vi "AutoCal.vi"(9 "Std Devs":dbl=1.0, 10 "Target Color":enum16{"Red", "Green", "Blue"}(ring), 11 "Color Image":T1) -> (1 "Luminance Info":T2, 2 "Saturation Info":T2, 3 "Hue Info":T2, 5 "Number of Particles":i32)   [LabVIEW 2013]
uses:
  <vilib>/vision/Image Controls.llb/IMAQ Image.ctl
  <vilib>/vision/NI_Vision_Development_Module.lvlib
panel:
  in  "Manual":bool
  out "Original":T1(plugin-control)
  out "Lum Std Dev":sgl format="%.2f"
  out "Lum Mean":sgl format="%.2f"
  out "Sat Std Dev":sgl format="%.2f"
  out "Sat Mean":sgl format="%.2f"
  out "Hue Std Dev":sgl format="%.2f"
  out "Hue Mean":sgl format="%.2f"
  out "Waveform Graph 2":T3(graph)
  out "Search Color Standard  Dev":sgl format="%.2f"
  out "Search Color Mean":sgl format="%.2f"
  out "Waveform Graph":T4(graph)
  out "Image":T1(plugin-control)
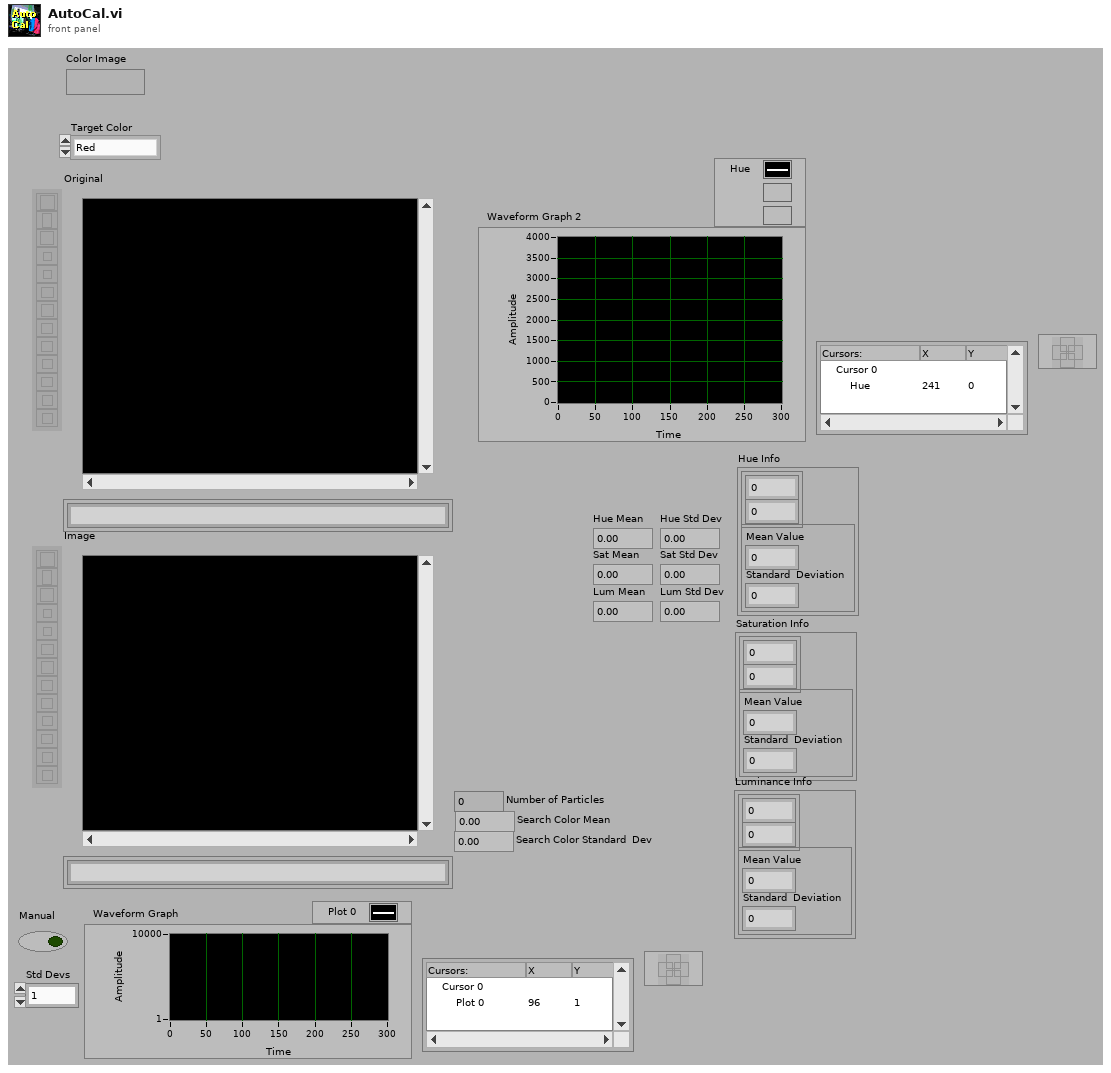
[diagram p1: front panel]
types:
  T1 = typedef "IMAQ Image.ctl" = refnum<image>
  T2 = cluster{cluster{sgl, sgl}, cluster{"Mean Value":sgl, "Standard  Deviation":sgl}}
  T3 = cluster{"Starting Value":sgl, "Incremental Value":sgl, "Histogram":u32[]}[]
  T4 = cluster{"Starting Value":sgl, "Incremental Value":sgl, "Histogram":u32[]}
  T5 = cluster{"Mean Value":sgl, "Standard  Deviation":sgl}
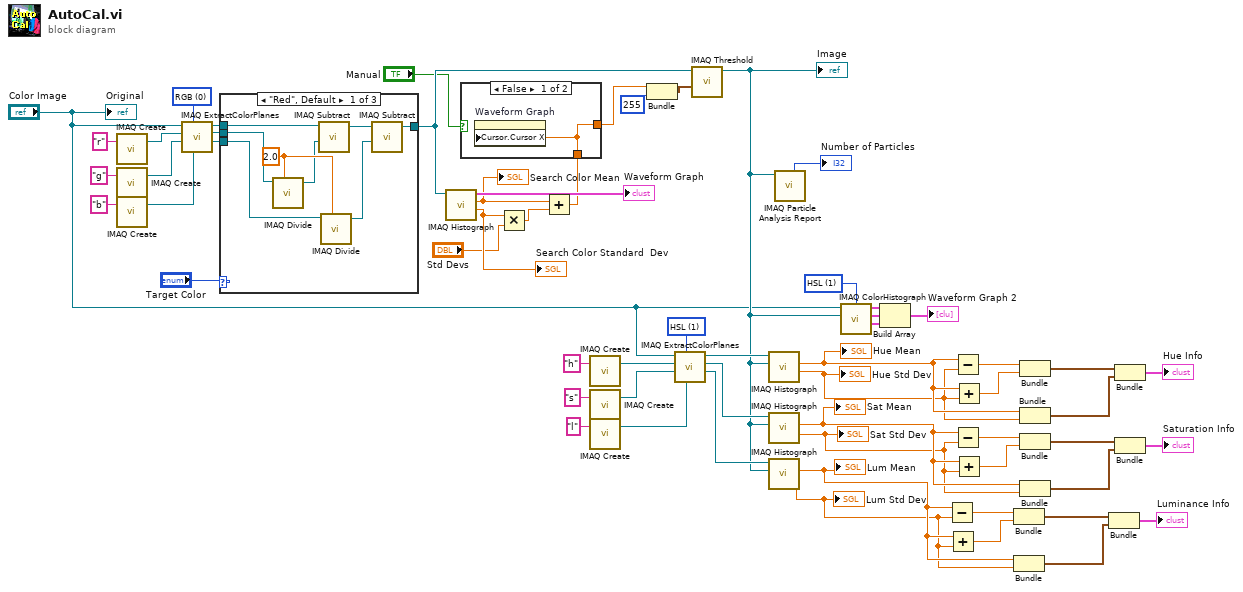
[diagram p0: block diagram]
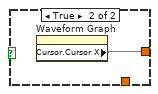
[diagram p2: hidden frame]
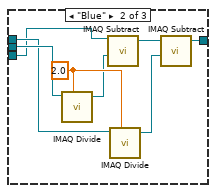
[diagram p3: hidden frame]
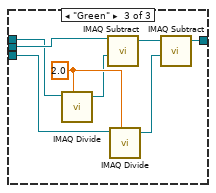
[diagram p4: hidden frame]
diagram:
  w42 = u16 1 items=["RGB", "HSL", "HSV", "HSI"] ("Color Mode")
  w47 = u16 1 items=["RGB", "HSL", "HSV", "HSI"] ("Color Mode")
  w55 = u16 0 items=["RGB", "HSL", "HSV", "HSI"] ("Color Mode")
  n1 = call "IMAQ Create"("Image Name"="r") -> ("New Image"=w58:T1)  [unwired: 3 in, 2 out]
  n2 = call "IMAQ Create"("Image Name"="g") -> ("New Image"=w57:T1)  [unwired: 3 in, 2 out]
  n3 = call "IMAQ Create"("Image Name"="b") -> ("New Image"=w56:T1)  [unwired: 3 in, 2 out]
  n4 = call "IMAQ ExtractColorPlanes"("Blue or Luma or Val or Inten Plane"=w56, "Color Mode"=w55, "Green or Sat Plane"=w57, "Red or Hue Plane"=w58, "Image Src"="Color Image") -> ("Blue or Luma or Val or Inten Plane out"=w53:T1, "Green or Sat Plane out"=w54:T1, "Red or Hue Plane out"=w52:T1)  [unwired: 1 in, 3 out]
  n5 = case shown="\"Red\", Default" "Target Color" {
    tunnel: w54 -> [w68 w72 w79]
    tunnel: w53 -> [w67 w70 w84]
    tunnel: w52 -> [w65 w71 w78]
    tunnel: [w62 w73 w80] -> w32
    frame "Red", Default {
      w66 = sgl 2.0 ("Constant")
      n6 = call "IMAQ Divide"("Image Src A"=w68, "Constant"=w66) -> ("Image Dst Out"=w64:T1)  [unwired: 4 in, 2 out]
      n7 = call "IMAQ Subtract"("Image Src A"=w65, "Image Src B"=w64) -> ("Image Dst Out"=w69:T1)  [unwired: 3 in, 3 out]
      n8 = call "IMAQ Divide"("Image Src A"=w67, "Constant"=w66) -> ("Image Dst Out"=w63:T1)  [unwired: 4 in, 2 out]
      n9 = call "IMAQ Subtract"("Image Src A"=w69, "Image Src B"=w63) -> ("Image Dst Out"=w62:T1)  [unwired: 3 in, 3 out]
    }
    frame "Blue" {
      w76 = sgl 2.0 ("Constant")
      n10 = call "IMAQ Divide"("Image Src A"=w72, "Constant"=w76) -> ("Image Dst Out"=w75:T1)  [unwired: 4 in, 2 out]
      n11 = call "IMAQ Subtract"("Image Src A"=w70, "Image Src B"=w75) -> ("Image Dst Out"=w77:T1)  [unwired: 3 in, 3 out]
      n12 = call "IMAQ Divide"("Image Src A"=w71, "Constant"=w76) -> ("Image Dst Out"=w74:T1)  [unwired: 4 in, 2 out]
      n13 = call "IMAQ Subtract"("Image Src A"=w77, "Image Src B"=w74) -> ("Image Dst Out"=w73:T1)  [unwired: 3 in, 3 out]
    }
    frame "Green" {
      w83 = sgl 2.0 ("Constant")
      n14 = call "IMAQ Divide"("Image Src A"=w78, "Constant"=w83) -> ("Image Dst Out"=w82:T1)  [unwired: 4 in, 2 out]
      n15 = call "IMAQ Subtract"("Image Src A"=w79, "Image Src B"=w82) -> ("Image Dst Out"=w85:T1)  [unwired: 3 in, 3 out]
      n16 = call "IMAQ Divide"("Image Src A"=w84, "Constant"=w83) -> ("Image Dst Out"=w81:T1)  [unwired: 4 in, 2 out]
      n17 = call "IMAQ Subtract"("Image Src A"=w85, "Image Src B"=w81) -> ("Image Dst Out"=w80:T1)  [unwired: 3 in, 3 out]
    }
  }
  n18 = call "IMAQ Histograph"("Image"=w32) -> ("Standard  Deviation"=w25:sgl, "Mean Value"=w48:sgl, "Histogram Graph"=→"Waveform Graph":T4)  [unwired: 4 in, 4 out]
  "Search Color Mean" <- w48
  "Search Color Standard  Dev" <- w25
  n19 = Multiply(x=w25, y="Std Devs") -> (x*y=w24:dbl)
  n20 = Add(x=w48, y=w24) -> (x+y=w26:dbl)
  n21 = case shown="False" "Manual" {
    tunnel: [w86 w87] -> w28
    tunnel: w26 -> [w86 _]
    frame False {
      n22 = property on="Waveform Graph" class="WFGraph (strict)"("Cursor.Cursor X"=w86) -> ()  [unwired: 2 in, 2 out]
    }
    frame True {
      n23 = property on="Waveform Graph" class="WFGraph (strict)"() -> ("Cursor.Cursor X"=w87:dbl)  [unwired: 2 in, 2 out]
    }
  }
  n24 = call "IMAQ Create"("Image Name"="h") -> ("New Image"=w38:T1)  [unwired: 3 in, 2 out]
  n25 = call "IMAQ Create"("Image Name"="s") -> ("New Image"=w37:T1)  [unwired: 3 in, 2 out]
  n26 = call "IMAQ Create"("Image Name"="l") -> ("New Image"=w36:T1)  [unwired: 3 in, 2 out]
  n27 = Bundle("Cursor.Cursor X"=w28, 255) -> (w49:cluster{"Cursor.Cursor X":dbl, i32})  [unwired: 1 out]
  n28 = call "IMAQ ExtractColorPlanes"("Blue or Luma or Val or Inten Plane"=w36, "Color Mode"=w42, "Green or Sat Plane"=w37, "Red or Hue Plane"=w38, "Image Src"="Color Image") -> ("Blue or Luma or Val or Inten Plane out"=w33:T1, "Green or Sat Plane out"=w34:T1, "Red or Hue Plane out"=w35:T1)  [unwired: 1 in, 3 out]
  n29 = call "IMAQ Threshold"("Range"=w49, "Image Src"=w32) -> ("Image Dst Out"=w27:T1)  [unwired: 4 in, 5 out]
  "Image" <- w27
  n30 = call "IMAQ Histograph"("Image Mask"=w27, "Image"=w35) -> ("Standard  Deviation"=w19:sgl, "Mean Value"=w20:sgl)  [unwired: 3 in, 5 out]
  "Hue Mean" <- w20
  "Hue Std Dev" <- w19
  n31 = call "IMAQ Histograph"("Image Mask"=w27, "Image"=w34) -> ("Standard  Deviation"=w7:sgl, "Mean Value"=w8:sgl)  [unwired: 3 in, 5 out]
  "Sat Mean" <- w8
  "Sat Std Dev" <- w7
  n32 = call "IMAQ Histograph"("Image Mask"=w27, "Image"=w33) -> ("Standard  Deviation"=w5:sgl, "Mean Value"=w6:sgl)  [unwired: 3 in, 5 out]
  "Lum Mean" <- w6
  "Lum Std Dev" <- w5
  n33 = call "IMAQ Particle Analysis Report"("Image"=w27) -> ("Number of Particles"=→"Number of Particles":i32)  [unwired: 2 in, 8 out]
  n34 = call "IMAQ ColorHistograph"("Color Mode"=w47, "Image Src"="Color Image", "Image Mask"=w27) -> ("Red or Hue Histogram Graph"=w46:T4, "Green or Sat Histogram Graph"=w45:T4, "Blue or Luma or Val or Inten Histogram Graph"=w44:T4)  [unwired: 2 in, 2 out]
  n35 = Build Array(w46, w45, w44) -> (→"Waveform Graph 2":T3)
  n36 = Subtract(x=w6, y=w5) -> (x-y=w12:sgl)
  n37 = Add(x=w6, y=w5) -> (x+y=w11:sgl)
  n38 = Subtract(x=w20, y=w19) -> (x-y=w22:sgl)
  n39 = Subtract(x=w8, y=w7) -> (x-y=w13:sgl)
  n40 = Add(x=w20, y=w19) -> (x+y=w21:sgl)
  n41 = Add(x=w8, y=w7) -> (x+y=w14:sgl)
  n42 = Bundle(w12, w11) -> (w10:cluster{sgl, sgl})  [unwired: 1 out]
  n43 = Bundle("Mean Value"=w6, "Standard  Deviation"=w5) -> (w9:T5)  [unwired: 1 out]
  n44 = Bundle(w22, w21) -> (w18:cluster{sgl, sgl})  [unwired: 1 out]
  n45 = Bundle("Mean Value"=w20, "Standard  Deviation"=w19) -> (w17:T5)  [unwired: 1 out]
  n46 = Bundle(w13, w14) -> (w15:cluster{sgl, sgl})  [unwired: 1 out]
  n47 = Bundle("Mean Value"=w8, "Standard  Deviation"=w7) -> (w16:T5)  [unwired: 1 out]
  n48 = Bundle(w10, w9) -> (→"Luminance Info":T2)  [unwired: 1 out]
  n49 = Bundle(w18, w17) -> (→"Hue Info":T2)  [unwired: 1 out]
  n50 = Bundle(w15, w16) -> (→"Saturation Info":T2)  [unwired: 1 out]
  "Original" <- "Color Image"
